vi "Global-force.vi"() -> ()   [LabVIEW 2020]
panel:
  out "golbal force":dbl
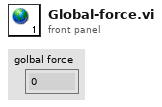
[diagram p1: front panel]
diagram:
